vi "rsscope_core_global.vi"() -> ()   [LabVIEW 2018] (continued)
, "Data Type"=0, "Command"="BUS{SerialBus}:CXPI:IFS:MAX", "Access"=2, "Range Table"="RsScope_rngCXPIExpectedIFSMax", "Read Callback"="", "Write Callback"="", "Supported Models"="", "Instrument Options"="K76", "Flags"=0, "Help"="Sets the maximum for the inter-frame-space range.\n\nAvailable Repeated Capabilities:\nSerialBus: SB1, SB2, SB3, SB4\r\n\nRemote-control command(s):\nBUS<m>:CXPI:IFS:MAX"}, {"Level"=3, "Class Only"=TRUE, "Identifier"="", "Descriptive Name"="Decoding Results", "Data Type"=0, "Command"="", "Access"=0, "Range Table"="", "Read Callback"="", "Write Callback"="", "Supported Models"="", "Instrument Options"="", "Flags"=0, "Help"="Returns the CXPI decoding results."}, {"Level"=4, "Class Only"=FALSE, "Identifier"="RSSCOPE_ATTR_PROTOCOL_CXPI_FRAME_COUNT", "Descriptive Name"="Protocol CXPI Frame Count", "Data Type"=0, "Command"="BUS{SerialBus}:CXPI:RES:FCO?", "Access"=0, "Range Table"="", "Read Callback"="", "Write Callback"="", "Supported Models"="", "Instrument Options"="K76", "Flags"=0, "Help"="Returns the number of frames in the acquisition.\n\nAvailable Repeated Capabilities:\nSerialBus: SB1, SB2, SB3, SB4\r\n\nRemote-control command(s):\nBUS<m>:CXPI:RESult:FCOunt?"}, {"Level"=2, "Class Only"=TRUE, "Identifier"="", "Descriptive Name"="PCIe", "Data Type"=0, "Command"="", "Access"=0, "Range Table"="", "Read Callback"="", "Write Callback"="", "Supported Models"="", "Instrument Options"="", "Flags"=0, "Help"="R&S RTO-K72 is a firmware option that enables the R&S RTO to analyze Peripheral Component Interconnect Express (PCIe) signals encoded by the PCIe standard, generation 1 and 2."}, {"Level"=3, "Class Only"=FALSE, "Identifier"="RSSCOPE_ATTR_PROTOCOL_PCIE_GENERATION", "Descriptive Name"="Protocol PCIe Generation", "Data Type"=0, "Command"="BUS{SerialBus}:PCIE:GEN", "Access"=2, "Range Table"="RsScope_rngPCIeGeneration", "Read Callback"="", "Write Callback"="", "Supported Models"="", "Instrument Options"="", "Flags"=0, "Help"="Selects the generation of the PCIe technology.\n\nAvailable Repeated Capabilities:\nSerialBus: SB1, SB2, SB3, SB4\r\n\nRemote-control command(s):\nBUS<m>:PCIE:GEN"}, {"Level"=3, "Class Only"=FALSE, "Identifier"="RSSCOPE_ATTR_PROTOCOL_PCIE_LINK", "Descriptive Name"="Protocol PCIe Link", "Data Type"=0, "Command"="BUS{SerialBus}:PCIE:LNKW", "Access"=2, "Range Table"="RsScope_rngPCIeLink", "Read Callback"="", "Write Callback"="", "Supported Models"="", "Instrument Options"="K72", "Flags"=0, "Help"="Selects the link width, the number of lanes that are used for the transmission of the data.\n\nAvailable Repeated Capabilities:\nSerialBus: SB1, SB2, SB3, SB4\r\n\nRemote-control command(s):\nBUS<m>:PCIE:LNKW"}, {"Level"=3, "Class Only"=FALSE, "Identifier"="RSSCOPE_ATTR_PROTOCOL_PCIE_DESCRAMBLING", "Descriptive Name"="Protocol PCIe Descrambling", "Data Type"=3, "Command"="BUS{SerialBus}:PCIE:DSCR", "Access"=2, "Range Table"="", "Read Callback"="", "Write Callback"="", "Supported Models"="", "Instrument Options"="K72", "Flags"=0, "Help"="Enables descrambling of the data.\n\nAvailable Repeated Capabilities:\nSerialBus: SB1, SB2, SB3, SB4\r\n\nRemote-control command(s):\nBUS<m>:PCIE:DSCRambling"}, {"Level"=3, "Class Only"=FALSE, "Identifier"="RSSCOPE_ATTR_PROTOCOL_PCIE_FILTER_IDLE", "Descriptive Name"="Protocol PCIe Filter Idle", "Data Type"=3, "Command"="BUS{SerialBus}:PCIE:FIDL", "Access"=2, "Range Table"="", "Read Callback"="", "Write Callback"="", "Supported Models"="", "Instrument Options"="K72", "Flags"=0, "Help"="Enables the filtering of idle packets.\n\nAvailable Repeated Capabilities:\nSerialBus: SB1, SB2, SB3, SB4\r\n\nRemote-control command(s):\nBUS<m>:PCIE:FIDLe"}, {"Level"=3, "Class Only"=FALSE, "Identifier"="RSSCOPE_ATTR_PROTOCOL_PCIE_SHOW_MULTIPLE_LANES", "Descriptive Name"="Protocol PCIe Show Multiple Lanes", "Data Type"=3, "Command"="BUS{SerialBus}:PCIE:SML", "Access"=2, "Range Table"="", "Read Callback"="", "Write Callback"="", "Supported Models"="", "Instrument Options"="K72", "Flags"=0, "Help"="Enables the display of the result in multiple lanes.\n\nAvailable Repeated Capabilities:\nSerialBus: SB1, SB2, SB3, SB4\r\n\nRemote-control command(s):\nBUS<m>:PCIE:SMLanes"}, {"Level"=3, "Class Only"=TRUE, "Identifier"="", "Descriptive Name"="Lane", "Data Type"=0, "Command"="", "Access"=0, "Range Table"="", "Read Callback"="", "Write Callback"="", "Supported Models"="", "Instrument Options"="", "Flags"=0, "Help"="Class for Lane repcap."}, {"Level"=4, "Class Only"=FALSE, "Identifier"="RSSCOPE_ATTR_PROTOCOL_PCIE_SOURCE_LANE_ZERO", "Descriptive Name"="Protocol PCIe Source Lane Zero", "Data Type"=0, "Command"="BUS{SerialBus}:PCIE:LZER:SOUR", "Access"=2, "Range Table"="rsscope_rngProtocolWaveformSource", "Read Callback"="", "Write Callback"="", "Supported Models"="", "Instrument Options"="K72", "Flags"=0, "Help"="Sets the signal sources for Lane 0.\n\nAvailable Repeated Capabilities:\nSerialBus: SB1, SB2, SB3, SB4\r\n\nRemote-control command(s):\nBUS<m>:PCIE:LZER:SOURce"}, {"Level"=4, "Class Only"=FALSE, "Identifier"="RSSCOPE_ATTR_PROTOCOL_PCIE_SOURCE_LANE_ONE", "Descriptive Name"="Protocol PCIe Source Lane One", "Data Type"=0, "Command"="BUS{SerialBus}:PCIE:LONE:SOUR", "Access"=2, "Range Table"="rsscope_rngProtocolWaveformSource", "Read Callback"="", "Write Callback"="", "Supported Models"="", "Instrument Options"="K72", "Flags"=0, "Help"="Sets the signal sources for the corresponding logical lane.\n\nAvailable Repeated Capabilities:\nSerialBus: SB1, SB2, SB3, SB4\r\n\nRemote-control command(s):\nBUS<m>:PCIE:LONE:SOURce"}, {"Level"=4, "Class Only"=FALSE, "Identifier"="RSSCOPE_ATTR_PROTOCOL_PCIE_SOURCE_LANE_TWO", "Descriptive Name"="Protocol PCIe Source Lane Two", "Data Type"=0, "Command"="BUS{SerialBus}:PCIE:LTWO:SOUR", "Access"=2, "Range Table"="rsscope_rngProtocolWaveformSource", "Read Callback"="", "Write Callback"="", "Supported Models"="", "Instrument Options"="K72", "Flags"=0, "Help"="Sets the signal sources for the corresponding logical lane.\n\nAvailable Repeated Capabilities:\nSerialBus: SB1, SB2, SB3, SB4\r\n\nRemote-control command(s):\nBUS<m>:PCIE:LTWO:SOURce"}, {"Level"=4, "Class Only"=FALSE, "Identifier"="RSSCOPE_ATTR_PROTOCOL_PCIE_SOURCE_LANE_THREE", "Descriptive Name"="Protocol PCIe Source Lane Three", "Data Type"=0, "Command"="BUS{SerialBus}:PCIE:LTHR:SOUR", "Access"=2, "Range Table"="rsscope_rngProtocolWaveformSource", "Read Callback"="", "Write Callback"="", "Supported Models"="", "Instrument Options"="K72", "Flags"=0, "Help"="Sets the signal sources for the corresponding logical lane.\n\nAvailable Repeated Capabilities:\nSerialBus: SB1, SB2, SB3, SB4\r\n\nRemote-control command(s):\nBUS<m>:PCIE:LTHRee:SOURce"}, {"Level"=4, "Class Only"=FALSE, "Identifier"="RSSCOPE_ATTR_PROTOCOL_PCIE_THRESHOLD_LOW_LANE_ZERO", "Descriptive Name"="Protocol PCIe Threshold Low Lane Zero", "Data Type"=1, "Command"="BUS{SerialBus}:PCIE:LZER:THRL", "Access"=2, "Range Table"="RsScope_rngPCIeThreshold", "Read Callback"="", "Write Callback"="", "Supported Models"="", "Instrument Options"="K72", "Flags"=0, "Help"="Sets the lower threshold value for the respective lane.\n\nAvailable Repeated Capabilities:\nSerialBus: SB1, SB2, SB3, SB4\r\n\nRemote-control command(s):\nBUS<m>:PCIE:LZER:THRLow"}, {"Level"=4, "Class Only"=FALSE, "Identifier"="RSSCOPE_ATTR_PROTOCOL_PCIE_THRESHOLD_LOW_LANE_ONE", "Descriptive Name"="Protocol PCIe Threshold Low Lane One", "Data Type"=1, "Command"="BUS{SerialBus}:PCIE:LONE:THRL", "Access"=2, "Range Table"="RsScope_rngPCIeThreshold", "Read Callback"="", "Write Callback"="", "Supported Models"="", "Instrument Options"="K72", "Flags"=0, "Help"="Sets the lower threshold value for the respective lane.\n\nAvailable Repeated Capabilities:\nSerialBus: SB1, SB2, SB3, SB4\r\n\nRemote-control command(s):\nBUS<m>:PCIE:LONE:THRLow"}, {"Level"=4, "Class Only"=FALSE, "Identifier"="RSSCOPE_ATTR_PROTOCOL_PCIE_THRESHOLD_LOW_LANE_TWO", "Descriptive Name"="Protocol PCIe Threshold Low Lane Two", "Data Type"=1, "Command"="BUS{SerialBus}:PCIE:LTWO:THRL", "Access"=2, "Range Table"="RsScope_rngPCIeThreshold", "Read Callback"="", "Write Callback"="", "Supported Models"="", "Instrument Options"="K72", "Flags"=0, "Help"="Sets the lower threshold value for the respective lane.\n\nAvailable Repeated Capabilities:\nSerialBus: SB1, SB2, SB3, SB4\r\n\nRemote-control command(s):\nBUS<m>:PCIE:LTWO:THRLow"}, {"Level"=4, "Class Only"=FALSE, "Identifier"="RSSCOPE_ATTR_PROTOCOL_PCIE_THRESHOLD_LOW_LANE_THREE", "Descriptive Name"="Protocol PCIe Threshold Low Lane Three", "Data Type"=1, "Command"="BUS{SerialBus}:PCIE:LTHR:THRL", "Access"=2, "Range Table"="RsScope_rngPCIeThreshold", "Read Callback"="", "Write Callback"="", "Supported Models"="", "Instrument Options"="K72", "Flags"=0, "Help"="Sets the lower threshold value for the respective lane.\n\nAvailable Repeated Capabilities:\nSerialBus: SB1, SB2, SB3, SB4\r\n\nRemote-control command(s):\nBUS<m>:PCIE:LTHRee:THRLow"}, {"Level"=4, "Class Only"=FALSE, "Identifier"="RSSCOPE_ATTR_PROTOCOL_PCIE_THRESHOLD_HIGH_LANE_ZERO", "Descriptive Name"="Protocol PCIe Threshold High Lane Zero", "Data Type"=1, "Command"="BUS{SerialBus}:PCIE:LZER:THRH", "Access"=2, "Range Table"="RsScope_rngPCIeThreshold", "Read Callback"="", "Write Callback"="", "Supported Models"="", "Instrument Options"="K72", "Flags"=0, "Help"="Sets the high threshold value for the respective lane.\n\nAvailable Repeated Capabilities:\nSerialBus: SB1, SB2, SB3, SB4\r\n\nRemote-control command(s):\nBUS<m>:PCIE:LZER:THRHigh"}, {"Level"=4, "Class Only"=FALSE, "Identifier"="RSSCOPE_ATTR_PROTOCOL_PCIE_THRESHOLD_HIGH_LANE_ONE", "Descriptive Name"="Protocol PCIe Threshold High Lane One", "Data Type"=1, "Command"="BUS{SerialBus}:PCIE:LONE:THRH", "Access"=2, "Range Table"="RsScope_rngPCIeThreshold", "Read Callback"="", "Write Callback"="", "Supported Models"="", "Instrument Options"="K72", "Flags"=0, "Help"="Sets the high threshold value for the respective lane.\n\nAvailable Repeated Capabilities:\nSerialBus: SB1, SB2, SB3, SB4\r\n\nRemote-control command(s):\nBUS<m>:PCIE:LONE:THRHigh"}, {"Level"=4, "Class Only"=FALSE, "Identifier"="RSSCOPE_ATTR_PROTOCOL_PCIE_THRESHOLD_HIGH_LANE_TWO", "Descriptive Name"="Protocol PCIe Threshold High Lane Two", "Data Type"=1, "Command"="BUS{SerialBus}:PCIE:LTWO:THRH", "Access"=2, "Range Table"="RsScope_rngPCIeThreshold", "Read Callback"="", "Write Callback"="", "Supported Models"="", "Instrument Options"="K72", "Flags"=0, "Help"="Sets the high threshold value for the respective lane.\n\nAvailable Repeated Capabilities:\nSerialBus: SB1, SB2, SB3, SB4\r\n\nRemote-control command(s):\nBUS<m>:PCIE:LTWO:THRHigh"}, {"Level"=4, "Class Only"=FALSE, "Identifier"="RSSCOPE_ATTR_PROTOCOL_PCIE_THRESHOLD_HIGH_LANE_THREE", "Descriptive Name"="Protocol PCIe Threshold High Lane Three", "Data Type"=1, "Command"="BUS{SerialBus}:PCIE:LTHR:THRH", "Access"=2, "Range Table"="RsScope_rngPCIeThreshold", "Read Callback"="", "Write Callback"="", "Supported Models"="", "Instrument Options"="K72", "Flags"=0, "Help"="Sets the high threshold value for the respective lane.\n\nAvailable Repeated Capabilities:\nSerialBus: SB1, SB2, SB3, SB4\r\n\nRemote-control command(s):\nBUS<m>:PCIE:LTHRee:THRHigh"}, {"Level"=3, "Class Only"=TRUE, "Identifier"="", "Descriptive Name"="CDR", "Data Type"=0, "Command"="", "Access"=0, "Range Table"="", "Read Callback"="", "Write Callback"="", "Supported Models"="", "Instrument Options"="", "Flags"=0, "Help"="The process of clock data recovery (CDR) generates a reference clock from a highspeed serial data stream that is sent without a dedicated clock signal. The generated clock signal matches the frequency and is aligned to the phase of the data stream. The recovered clock can be used to sample the data stream and to obtain the sequence of transmitted bits."}, {"Level"=4, "Class Only"=FALSE, "Identifier"="RSSCOPE_ATTR_PROTOCOL_PCIE_CDR_NOMINAL_BITRATE", "Descriptive Name"="Protocol PCIe CDR Nominal Bitrate", "Data Type"=5, "Command"="BUS{SerialBus}:CDR:BITR", "Access"=2, "Range Table"="RsScope_rngPCIeCDRNominalBitrate", "Read Callback"="", "Write Callback"="", "Supported Models"="", "Instrument Options"="K72", "Flags"=0, "Help"="Sets the quiescent frequency of the PLL. It corresponds to the data rate of the data stream from which the clock is to be recovered.\n\nAvailable Repeated Capabilities:\nSerialBus: SB1, SB2, SB3, SB4\r\n\nRemote-control command(s):\nBUS<m>:CDR:BITRate"}, {"Level"=4, "Class Only"=FALSE, "Identifier"="RSSCOPE_ATTR_PROTOCOL_PCIE_CDR_PLL_ORDER", "Descriptive Name"="Protocol PCIe CDR PLL Order", "Data Type"=0, "Command"="BUS{SerialBus}:CDR:PLL:ORD", "Access"=2, "Range Table"="RsScope_rngPCIeCDRPLLOrder", "Read Callback"="", "Write Callback"="", "Supported Models"="", "Instrument Options"="K72", "Flags"=0, "Help"="Sets the order of the PLL: first or second order. PLL of higher order can compensate for more complex jitter behavior.\n\nAvailable Repeated Capabilities:\nSerialBus: SB1, SB2, SB3, SB4\r\n\nRemote-control command(s):\nBUS<m>:CDR:PLL:ORDer"}, {"Level"=4, "Class Only"=FALSE, "Identifier"="RSSCOPE_ATTR_PROTOCOL_PCIE_CDR_PLL_BANDWIDTH", "Descriptive Name"="Protocol PCIe CDR PLL Bandwidth", "Data Type"=1, "Command"="BUS{SerialBus}:CDR:PLL:BWID", "Access"=2, "Range Table"="", "Read Callback"="", "Write Callback"="", "Supported Models"="", "Instrument Options"="K72", "Flags"=0, "Help"="Sets the PLL bandwidth. It defines the part of the spectrum that the PLL can follow during synchronization. The PLL bandwidth is usually defined by the transmission standard.\n\nAvailable Repeated Capabilities:\nSerialBus: SB1, SB2, SB3, SB4\r\n\nRemote-control command(s):\nBUS<m>:CDR:PLL:BWIDth"}, {"Level"=4, "Class Only"=FALSE, "Identifier"="RSSCOPE_ATTR_PROTOCOL_PCIE_CDR_PLL_RELATIVE_BANDWIDTH", "Descriptive Name"="Protocol PCIe CDR PLL Relative Bandwidth", "Data Type"=1, "Command"="BUS{SerialBus}:CDR:PLL:RELB", "Access"=2, "Range Table"="RsScope_rngPCIeCDRPLLRelativeBandwidth", "Read Callback"="", "Write Callback"="", "Supported Models"="", "Instrument Options"="K72", "Flags"=0, "Help"="Sets the PLL bandwidth. It defines the part of the spectrum that the PLL can follow during synchronization. The PLL bandwidth is usually defined by the transmission standard.\n\nAvailable Repeated Capabilities:\nSerialBus: SB1, SB2, SB3, SB4\r\n\nRemote-control command(s):\nBUS<m>:CDR:PLL:RELBwidth"}, {"Level"=4, "Class Only"=FALSE, "Identifier"="RSSCOPE_ATTR_PROTOCOL_PCIE_CDR_PLL_DAMPING", "Descriptive Name"="Protocol PCIe CDR PLL Damping", "Data Type"=1, "Command"="BUS{SerialBus}:CDR:PLL:DAMP", "Access"=2, "Range Table"="RsScope_rngPCIeCDRPLLDamping", "Read Callback"="", "Write Callback"="", "Supported Models"="", "Instrument Options"="K72", "Flags"=0, "Help"="Sets the damping factor, which is only relevant for second order PLL.\n\nAvailable Repeated Capabilities:\nSerialBus: SB1, SB2, SB3, SB4\r\n\nRemote-control command(s):\nBUS<m>:CDR:PLL:DAMPing"}, {"Level"=4, "Class Only"=FALSE, "Identifier"="RSSCOPE_ATTR_PROTOCOL_PCIE_CDR_INITIAL_PHASE_SYNC", "Descriptive Name"="Protocol PCIe CDR Initial Phase Sync", "Data Type"=0, "Command"="BUS{SerialBus}:CDR:SYNC", "Access"=2, "Range Table"="RsScope_rngPCIeCDRInitialPhaseSync", "Read Callback"="", "Write Callback"="", "Supported Models"="", "Instrument Options"="K72", "Flags"=0, "Help"="Defines the phase reference for the first clock edge.\n\nAvailable Repeated Capabilities:\nSerialBus: SB1, SB2, SB3, SB4\r\n\nRemote-control command(s):\nBUS<m>:CDR:SYNC"}, {"Level"=4, "Class Only"=FALSE, "Identifier"="RSSCOPE_ATTR_PROTOCOL_PCIE_CDR_SELECTED_RESULTS", "Descriptive Name"="Protocol PCIe CDR Selected Results", "Data Type"=0, "Command"="BUS{SerialBus}:CDR:RES", "Access"=2, "Range Table"="RsScope_rngPCIeCDRSelectedResults", "Read Callback"="", "Write Callback"="", "Supported Models"="", "Instrument Options"="K72", "Flags"=0, "Help"="The PLL requires some time to synchronize to the phase of the data stream. You can select when the CDR algorithm returns clock edges.\n\nAvailable Repeated Capabilities:\nSerialBus: SB1, SB2, SB3, SB4\r\n\nRemote-control command(s):\nBUS<m>:CDR:RESults"}, {"Level"=3, "Class Only"=TRUE, "Identifier"="", "Descriptive Name"="DSP", "Data Type"=0, "Command"="", "Access"=0, "Range Table"="", "Read Callback"="", "Write Callback"="", "Supported Models"="", "Instrument Options"="", "Flags"=0, "Help"="You can enable and define the equalization techniques used for the equalization at the reciever side of the signal."}, {"Level"=4, "Class Only"=TRUE, "Identifier"="", "Descriptive Name"="DFE", "Data Type"=0, "Command"="", "Access"=0, "Range Table"="", "Read Callback"="", "Write Callback"="", "Supported Models"="", "Instrument Options"="", "Flags"=0, "Help"="Defines the settings of the decision feedback equalization (DFE). DFE correction is needed when the channel is distosrted."}, {"Level"=5, "Class Only"=FALSE, "Identifier"="RSSCOPE_ATTR_PROTOCOL_PCIE_DSP_DFE_ENABLED", "Descriptive Name"="Protocol PCIe DSP DFE Enabled", "Data Type"=3, "Command"="BUS{SerialBus}:PCIE:DFE:ENBL", "Access"=2, "Range Table"="", "Read Callback"="", "Write Callback"="", "Supported Models"="", "Instrument Options"="K72", "Flags"=0, "Help"="Enables the use of the decision feedback equalization for PCIe.\n\nAvailable Repeated Capabilities:\nSerialBus: SB1, SB2, SB3, SB4\r\n\nRemote-control command(s):\nBUS<m>:PCIE:DFE:ENBLe"}, {"Level"=5, "Class Only"=FALSE, "Identifier"="RSSCOPE_ATTR_PROTOCOL_PCIE_DSP_DFE_ESTIMATE_COEFFICIENTS_ENABLED", "Descriptive Name"="Protocol PCIe DSP DFE Estimate Coefficients Enabled", "Data Type"=3, "Command"="BUS{SerialBus}:PCIE:DFE:AUTO", "Access"=2, "Range Table"="", "Read Callback"="", "Write Callback"="", "Supported Models"="", "Instrument Options"="K72", "Flags"=0, "Help"="Enables the use of estimate coefficients\n\nAvailable Repeated Capabilities:\nSerialBus: SB1, SB2, SB3, SB4\r\n\nRemote-control command(s):\nBUS<m>:PCIE:DFE:AUTO"}, {"Level"=5, "Class Only"=FALSE, "Identifier"="RSSCOPE_ATTR_PROTOCOL_PCIE_DSP_DFE_COEFFICIENT", "Descriptive Name"="Protocol PCIe DSP DFE Coefficient", "Data Type"=1, "Command"="BUS{SerialBus}:PCIE:DFE:COEF", "Access"=2, "Range Table"="RsScope_rngDSPDFECoefficient", "Read Callback"="", "Write Callback"="", "Supported Models"="", "Instrument Options"="K72", "Flags"=0, "Help"="Sets the value of the coefficient for the DFE.\n\nAvailable Repeated Capabilities:\nSerialBus: SB1, SB2, SB3, SB4\r\n\nRemote-control command(s):\nBUS<m>:PCIE:DFE:COEFficient"}, {"Level"=5, "Class Only"=FALSE, "Identifier"="RSSCOPE_ATTR_PROTOCOL_PCIE_DSP_DFE_NUMBER_OF_TAPS", "Descriptive Name"="Protocol PCIe DSP DFE Number Of Taps", "Data Type"=0, "Command"="BUS{SerialBus}:PCIE:DFE:TCON", "Access"=2, "Range Table"="RsScope_rngDSPDFENumberOfTaps", "Read Callback"="", "Write Callback"="", "Supported Models"="", "Instrument Options"="K72", "Flags"=0, "Help"="Sets a number of taps for the decision feedback filter.\n\nAvailable Repeated Capabilities:\nSerialBus: SB1, SB2, SB3, SB4\r\n\nRemote-control command(s):\nBUS<m>:PCIE:DFE:TCONt"}, {"Level"=3, "Class Only"=TRUE, "Identifier"="", "Descriptive Name"="Decoding Results", "Data Type"=0, "Command"="", "Access"=0, "Range Table"="", "Read Callback"="", "Write Callback"="", "Supported Models"="", "Instrument Options"="", "Flags"=0, "Help"="Returns the PCIe decoding results."}, {"Level"=4, "Class Only"=FALSE, "Identifier"="RSSCOPE_ATTR_PROTOCOL_PCIE_PACKET_COUNT", "Descriptive Name"="Protocol PCIe Packet Count", "Data Type"=0, "Command"="BUS{SerialBus}:PCIE:RES:PCO?", "Access"=0, "Range Table"="", "Read Callback"="", "Write Callback"="", "Supported Models"="RTO|RTP", "Instrument Options"="K72", "Flags"=0, "Help"="Returns the packet count for the selected serial bus, i.e. the number of packets in the present acquisition.\n\nAvailable Repeated Capabilities:\nSerialBus: SB1, SB2, SB3, SB4\r\n\nRemote-control command(s):\nBUS<m>:PCIE:RESult:PCOunt?"}, {"Level"=4, "Class Only"=FALSE, "Identifier"="RSSCOPE_ATTR_PROTOCOL_PCIE_SELECTED_PACKET", "Descriptive Name"="Protocol PCIe Selected Packet", "Data Type"=0, "Command"="", "Access"=2, "Range Table"="", "Read Callback"="", "Write Callback"="", "Supported Models"="", "Instrument Options"="", "Flags"=0, "Help"="Sets the selector for the Packet repeated capability.\n\nAvailable Repeated Capabilities:\nNone\n\nRemote-control command(s):\n"}, {"Level"=4, "Class Only"=FALSE, "Identifier"="RSSCOPE_ATTR_PROTOCOL_PCIE_PACKET_BIT_RATE", "Descriptive Name"="Protocol PCIe Packet Bit Rate", "Data Type"=5, "Command"="BUS{SerialBus}:PCIE:RES:PACK<Packet>:BITR?", "Access"=0, "Range Table"="", "Read Callback"="rsscope_FormatPCIePacketRepCapInt64_ReadCallback.vi", "Write Callback"="rsscope_FormatPCIePacketRepCapInt64_WriteCallback.vi", "Supported Models"="", "Instrument Options"="", "Flags"=0, "Help"="Returns the bit rate of the selected packet.\n\nAvailable Repeated Capabilities:\nSerialBus: SB1, SB2, SB3, SB4\r\n\nRemote-control command(s):\nBUS<m>:PCIE:RESult:PACKet<n>:BITRate?"}, {"Level"=2, "Class Only"=TRUE, "Identifier"="", "Descriptive Name"="DDR", "Data Type"=0, "Command"="", "Access"=0, "Range Table"="", "Read Callback"="", "Write Callback"="", "Supported Models"="", "Instrument Options"="", "Flags"=0, "Help"="Double Data Rate memory (DDR) is a type of Synchronous Dynamic Random Access Memory (SDRAM). Option R&S RTO-K91"}, {"Level"=3, "Class Only"=FALSE, "Identifier"="RSSCOPE_ATTR_PROTOCOL_DDR_STANDARD", "Descriptive Name"="Protocol DDR Standard", "Data Type"=0, "Command"="BUS{SerialBus}:DDR:STAN", "Access"=2, "Range Table"="RsScope_rngDDRStandard", "Read Callback"="", "Write Callback"="", "Supported Models"="", "Instrument Options"="K91|K93", "Flags"=0, "Help"="Selects the DDR standard.\n\nAvailable Repeated Capabilities:\nSerialBus: SB1, SB2, SB3, SB4\r\n\nRemote-control command(s):\nBUS<m>:DDR:STANdard"}, {"Level"=3, "Class Only"=FALSE, "Identifier"="RSSCOPE_ATTR_PROTOCOL_DDR_DATA_SOURCE", "Descriptive Name"="Protocol DDR Data Source", "Data Type"=0, "Command"="BUS{SerialBus}:DDR:DATA:SOUR", "Access"=2, "Range Table"="rsscope_rngProtocolDDRSource", "Read Callback"="", "Write Callback"="", "Supported Models"="", "Instrument Options"="K91|K93", "Flags"=0, "Help"="Selects the source for the data output signal.\n\nAvailable Repeated Capabilities:\nSerialBus: SB1, SB2, SB3, SB4\r\n\nRemote-control command(s):\nBUS<m>:DDR:DATA:SOURce"}, {"Level"=3, "Class Only"=FALSE, "Identifier"="RSSCOPE_ATTR_PROTOCOL_DDR_DATA_THRESHOLD", "Descriptive Name"="Protocol DDR Data Threshold", "Data Type"=1, "Command"="BUS{SerialBus}:DDR:DATA:THR", "Access"=2, "Range Table"="RsScope_rngProtocolDDRThreshold", "Read Callback"="", "Write Callback"="", "Supported Models"="", "Instrument Options"="K91|K93", "Flags"=0, "Help"="Sets the threshold value for the digitization of the data line.\n\nAvailable Repeated Capabilities:\nSerialBus: SB1, SB2, SB3, SB4\r\n\nRemote-control command(s):\nBUS<m>:DDR:DATA:THReshold"}, {"Level"=3, "Class Only"=FALSE, "Identifier"="RSSCOPE_ATTR_PROTOCOL_DDR_DATA_HYSTERESIS", "Descriptive Name"="Protocol DDR Data Hysteresis", "Data Type"=1, "Command"="BUS{SerialBus}:DDR:DATA:HYST", "Access"=2, "Range Table"="RsScope_rngProtocolDDRHysteresis", "Read Callback"="", "Write Callback"="", "Supported Models"="", "Instrument Options"="K91|K93", "Flags"=0, "Help"="Sets a value for the hysteresis of the data.\n\nAvailable Repeated Capabilities:\nSerialBus: SB1, SB2, SB3, SB4\r\n\nRemote-control command(s):\nBUS<m>:DDR:DATA:HYSTeresis"}, {"Level"=3, "Class Only"=FALSE, "Identifier"="RSSCOPE_ATTR_PROTOCOL_DDR_STROBE_SOURCE", "Descriptive Name"="Protocol DDR Strobe Source", "Data Type"=0, "Command"="BUS{SerialBus}:DDR:STRB:SOUR", "Access"=2, "Range Table"="rsscope_rngProtocolDDRSource", "Read Callback"="", "Write Callback"="", "Supported Models"="", "Instrument Options"="K91|K93", "Flags"=0, "Help"="Selects the source for the strobe signal.\n\nAvailable Repeated Capabilities:\nSerialBus: SB1, SB2, SB3, SB4\r\n\nRemote-control command(s):\nBUS<m>:DDR:STRBe:SOURce"}, {"Level"=3, "Class Only"=FALSE, "Identifier"="RSSCOPE_ATTR_PROTOCOL_DDR_STROBE_THRESHOLD", "Descriptive Name"="Protocol DDR Strobe Threshold", "Data Type"=1, "Command"="BUS{SerialBus}:DDR:STRB:THR", "Access"=2, "Range Table"="RsScope_rngProtocolDDRThreshold", "Read Callback"="", "Write Callback"="", "Supported Models"="", "Instrument Options"="K91|K93", "Flags"=0, "Help"="Sets the threshold value for the digitization of the strobe line.\n\nAvailable Repeated Capabilities:\nSerialBus: SB1, SB2, SB3, SB4\r\n\nRemote-control command(s):\nBUS<m>:DDR:STRBe:THReshold"}, {"Level"=3, "Class Only"=FALSE, "Identifier"="RSSCOPE_ATTR_PROTOCOL_DDR_STROBE_HYSTERESIS", "Descriptive Name"="Protocol DDR Strobe Hysteresis", "Data Type"=1, "Command"="BUS{SerialBus}:DDR:STRB:HYST", "Access"=2, "Range Table"="RsScope_rngProtocolDDRHysteresis", "Read Callback"="", "Write Callback"="", "Supported Models"="", "Instrument Options"="K91|K93", "Flags"=0, "Help"="Sets a value for the hysteresis of the strobe.\n\nAvailable Repeated Capabilities:\nSerialBus: SB1, SB2, SB3, SB4\r\n\nRemote-control command(s):\nBUS<m>:DDR:STRBe:HYSTeresis"}, {"Level"=3, "Class Only"=TRUE, "Identifier"="", "Descriptive Name"="Decoding Results", "Data Type"=0, "Command"="", "Access"=0, "Range Table"="", "Read Callback"="", "Write Callback"="", "Supported Models"="", "Instrument Options"="", "Flags"=0, "Help"="Returns the DDR decoding results."}, {"Level"=4, "Class Only"=FALSE, "Identifier"="RSSCOPE_ATTR_PROTOCOL_DDR_FRAME_COUNT", "Descriptive Name"="Protocol DDR Frame Count", "Data Type"=0, "Command"="BUS{SerialBus}:DDR:RES:FCO?", "Access"=0, "Range Table"="", "Read Callback"="", "Write Callback"="", "Supported Models"="", "Instrument Options"="K91|K93", "Flags"=0, "Help"="Returns the number of decoded frames in the selected serial bus.\n\nAvailable Repeated Capabilities:\nSerialBus: SB1, SB2, SB3, SB4\r\n\nRemote-control command(s):\nBUS<m>:DDR:RESult:FCOunt?"}, {"Level"=4, "Class Only"=FALSE, "Identifier"="RSSCOPE_ATTR_PROTOCOL_DDR_SELECTED_FRAME", "Descriptive Name"="Protocol DDR Selected Frame", "Data Type"=0, "Command"="", "Access"=2, "Range Table"="", "Read Callback"="", "Write Callback"="", "Supported Models"="", "Instrument Options"="", "Flags"=0, "Help"="Sets selector repeated capability Frame.\n\nAvailable Repeated Capabilities:\nNone\n\nRemote-control command(s):\n"}, {"Level"=4, "Class Only"=FALSE, "Identifier"="RSSCOPE_ATTR_PROTOCOL_DDR_FRAME_STATUS", "Descriptive Name"="Protocol DDR Frame Status", "Data Type"=0, "Command"="BUS{SerialBus}:DDR:RES:FRAM<Frame>:STAT?", "Access"=0, "Range Table"="RsScope_rngDDRFrameStatus", "Read Callback"="rsscope_FormatDDRFrameRepCapInt32_ReadCallback.vi", "Write Callback"="", "Supported Models"="", "Instrument Options"="K91|K93", "Flags"=0, "Help"="Returns the status of the frame with the selected frame number (for the selected serial bus).\n\nAvailable Repeated Capabilities:\nSerialBus: SB1, SB2, SB3, SB4\r\n\nRemote-control command(s):\nBUS<m>:DDR:RESult:FRAMe<n>:STATe?"}, {"Level"=4, "Class Only"=FALSE, "Identifier"="RSSCOPE_ATTR_PROTOCOL_DDR_FRAME_START_TIME", "Descriptive Name"="Protocol DDR Frame Start Time", "Data Type"=1, "Command"="BUS{SerialBus}:DDR:RES:FRAM<Frame>:STAR?", "Access"=0, "Range Table"="", "Read Callback"="rsscope_FormatDDRFrameRepCapReal64_ReadCallback.vi", "Write Callback"="", "Supported Models"="", "Instrument Options"="K91|K93", "Flags"=0, "Help"="Returns the start time of the frame with the selected frame number (for the selected serial bus).\n\nAvailable Repeated Capabilities:\nSerialBus: SB1, SB2, SB3, SB4\r\n\nRemote-control command(s):\nBUS<m>:DDR:RESult:FRAMe<n>:STARt?"}, {"Level"=4, "Class Only"=FALSE, "Identifier"="RSSCOPE_ATTR_PROTOCOL_DDR_FRAME_STOP_TIME", "Descriptive Name"="Protocol DDR Frame Stop Time", "Data Type"=1, "Command"="BUS{SerialBus}:DDR:RES:FRAM<Frame>:STOP?", "Access"=0, "Range Table"="", "Read Callback"="rsscope_FormatDDRFrameRepCapReal64_ReadCallback.vi", "Write Callback"="", "Supported Models"="", "Instrument Options"="K91|K93", "Flags"=0, "Help"="Returns the stop time of the frame with the selected frame number (for the selected serial bus).\n\nAvailable Repeated Capabilities:\nSerialBus: SB1, SB2, SB3, SB4\r\n\nRemote-control command(s):\nBUS<m>:DDR:RESult:FRAMe<n>:STOP?"}, {"Level"=4, "Class Only"=FALSE, "Identifier"="RSSCOPE_ATTR_PROTOCOL_DDR_FRAME_TYPE", "Descriptive Name"="Protocol DDR Frame Type", "Data Type"=0, "Command"="BUS{SerialBus}:DDR:RES:FRAM<Frame>:TYPE?", "Access"=0, "Range Table"="RsScope_rngProtocolDDRFrameType", "Read Callback"="rsscope_FormatDDRFrameRepCapInt32_ReadCallback.vi", "Write Callback"="", "Supported Models"="", "Instrument Options"="K91|K93", "Flags"=0, "Help"="Returns the frame type for the selected serial bus and frame number.\n\nAvailable Repeated Capabilities:\nSerialBus: SB1, SB2, SB3, SB4\r\n\nRemote-control command(s):\nBUS<m>:DDR:RESult:FRAMe<n>:TYPE?"}, {"Level"=4, "Class Only"=FALSE, "Identifier"="RSSCOPE_ATTR_PROTOCOL_DDR_FRAME_NUMBER_OF_WORDS", "Descriptive Name"="Protocol DDR Frame Number Of Words", "Data Type"=0, "Command"="BUS{SerialBus}:DDR:RES:FRAM<Frame>:NWRD?", "Access"=0, "Range Table"="", "Read Callback"="rsscope_FormatDDRFrameRepCapInt32_ReadCallback.vi", "Write Callback"="", "Supported Models"="", "Instrument Options"="K91|K93", "Flags"=0, "Help"="Returns the number of words for the selected serial bus and frame number.\n\nAvailable Repeated Capabilities:\nSerialBus: SB1, SB2, SB3, SB4\r\n\nRemote-control command(s):\nBUS<m>:DDR:RESult:FRAMe<n>:NWRDs?"}, {"Level"=4, "Class Only"=FALSE, "Identifier"="RSSCOPE_ATTR_PROTOCOL_DDR_SELECTED_FIELD", "Descriptive Name"="Protocol DDR Selected Field", "Data Type"=0, "Command"="", "Access"=2, "Range Table"="", "Read Callback"="", "Write Callback"="", "Supported Models"="", "Instrument Options"="", "Flags"=0, "Help"="Sets selector repeated capability Field.\n\nAvailable Repeated Capabilities:\nNone\n\nRemote-control command(s):\n"}, {"Level"=4, "Class Only"=FALSE, "Identifier"="RSSCOPE_ATTR_PROTOCOL_DDR_FRAME_FIELD_STATUS", "Descriptive Name"="Protocol DDR Frame Field Status", "Data Type"=0, "Command"="BUS{SerialBus}:DDR:RES:FRAM<Frame>:FLD<Field>:STAT?", "Access"=0, "Range Table"="RsScope_rngDDRFrameStatus", "Read Callback"="rsscope_FormatDDRFieldRepCapInt32_ReadCallback.vi", "Write Callback"="", "Supported Models"="", "Instrument Options"="K91|K93", "Flags"=0, "Help"="Returns the status of the field with the selected field number within the frame with the selected frame number (for the selected serial bus).\n\nAvailable Repeated Capabilities:\nSerialBus: SB1, SB2, SB3, SB4\r\n\nRemote-control command(s):\nBUS<m>:DDR:RESult:FRAMe<n>:FLD<o>:STATus?"}, {"Level"=4, "Class Only"=FALSE, "Identifier"="RSSCOPE_ATTR_PROTOCOL_DDR_FRAME_FIELD_START_TIME", "Descriptive Name"="Protocol DDR Frame Field Start Time", "Data Type"=1, "Command"="BUS{SerialBus}:DDR:RES:FRAM<Frame>:FLD<Field>:STAR?", "Access"=0, "Range Table"="", "Read Callback"="rsscope_FormatDDRFieldRepCapReal64_ReadCallback.vi", "Write Callback"="", "Supported Models"="", "Instrument Options"="K91|K93", "Flags"=0, "Help"="Returns the start time of the field with the selected field number within the frame with the selected frame number (for the selected serial bus).\n\nAvailable Repeated Capabilities:\nSerialBus: SB1, SB2, SB3, SB4\r\n\nRemote-control command(s):\nBUS<m>:DDR:RESult:FRAMe<n>:FLD<o>:STARt?"}, {"Level"=4, "Class Only"=FALSE, "Identifier"="RSSCOPE_ATTR_PROTOCOL_DDR_FRAME_FIELD_STOP_TIME", "Descriptive Name"="Protocol DDR Frame Field Stop Time", "Data Type"=1, "Command"="BUS{SerialBus}:DDR:RES:FRAM<Frame>:FLD<Field>:STOP?", "Access"=0, "Range Table"="", "Read Callback"="rsscope_FormatDDRFieldRepCapReal64_ReadCallback.vi", "Write Callback"="", "Supported Models"="", "Instrument Options"="K91|K93", "Flags"=0, "Help"="Returns the stop time of the field with the selected field number within the frame with the selected frame number (for the selected serial bus).\n\nAvailable Repeated Capabilities:\nSerialBus: SB1, SB2, SB3, SB4\r\n\nRemote-control command(s):\nBUS<m>:DDR:RESult:FRAMe<n>:FLD<o>:STOP?"}, {"Level"=4, "Class Only"=FALSE, "Identifier"="RSSCOPE_ATTR_PROTOCOL_DDR_FRAME_FIELD_VALUE", "Descriptive Name"="Protocol DDR Frame Field Value", "Data Type"=0, "Command"="BUS{SerialBus}:DDR:RES:FRAM<Frame>:FLD<Field>:VAL?", "Access"=0, "Range Table"="", "Read Callback"="rsscope_FormatDDRFieldRepCapInt32_ReadCallback.vi", "Write Callback"="", "Supported Models"="", "Instrument Options"="K91|K93", "Flags"=0, "Help"="Returns the value of the field with the selected field number within the frame with the selected frame number (for the selected serial bus).\n\nAvailable Repeated Capabilities:\nSerialBus: SB1, SB2, SB3, SB4\r\n\nRemote-control command(s):\nBUS<m>:DDR:RESult:FRAMe<n>:FLD<o>:VAL?"}, {"Level"=4, "Class Only"=FALSE, "Identifier"="RSSCOPE_ATTR_PROTOCOL_DDR_FRAME_FIELD_FORMATTED_VALUE", "Descriptive Name"="Protocol DDR Frame Field Formatted Value", "Data Type"=2, "Command"="BUS{SerialBus}:DDR:RES:FRAM<Frame>:FLD<Field>:FVAL?", "Access"=0, "Range Table"="", "Read Callback"="rsscope_FormatDDRFieldRepCapString_ReadCallback.vi", "Write Callback"="", "Supported Models"="", "Instrument Options"="K91|K93", "Flags"=0, "Help"="Returns the formatted value of the field with the selected field number within the frame with the selected frame number (for the selected serial bus).\n\nAvailable Repeated Capabilities:\nSerialBus: SB1, SB2, SB3, SB4\r\n\nRemote-control command(s):\nBUS<m>:DDR:RESult:FRAMe<n>:FLD<o>:FVAL?"}, {"Level"=3, "Class Only"=TRUE, "Identifier"="", "Descriptive Name"="Eye Diagram", "Data Type"=0, "Command"="", "Access"=0, "Range Table"="", "Read Callback"="", "Write Callback"="", "Supported Models"="", "Instrument Options"="", "Flags"=0, "Help"="This class contains attributes and functions that provide eye diagram setup."}, {"Level"=4, "Class Only"=TRUE, "Identifier"="", "Descriptive Name"="Setup", "Data Type"=0, "Command"="", "Access"=0, "Range Table"="", "Read Callback"="", "Write Callback"="", "Supported Models"="", "Instrument Options"="", "Flags"=0, "Help"="Configure the source, the timing reference, and horizontal scale settings of the eye diagram. The vertical scale of the eye diagram is coupled to the vertical scale of the data source."}, {"Level"=5, "Class Only"=FALSE, "Identifier"="RSSCOPE_ATTR_EYE_DIAGRAM_STATE", "Descriptive Name"="Eye Diagram State", "Data Type"=3, "Command"="EYE{EyeDiagram}", "Access"=2, "Range Table"="", "Read Callback"="", "Write Callback"="", "Supported Models"="", "Instrument Options"="K91|K93", "Flags"=0, "Help"="Activates or deactivates the eye diagram.\n\nAvailable Repeated Capabilities:\nEyeDiagram: ED1, ED2, ED3, ED4\r\n\nRemote-control command(s):\nEYE<m>[:STATe]"}, {"Level"=5, "Class Only"=FALSE, "Identifier"="RSSCOPE_ATTR_EYE_DIAGRAM_SOURCE", "Descriptive Name"="Eye Diagram Source", "Data Type"=0, "Command"="EYE{EyeDiagram}:SOUR", "Access"=2, "Range Table"="rsscope_rngEyeDiagramSource", "Read Callback"="", "Write Callback"="", "Supported Models"="", "Instrument Options"="K91|K93", "Flags"=0, "Help"="Selects the waveform from which the eye diagram is generated (data source). For analog channels, peak detect, envelope, and average waveforms are not supported.\n\nAvailable Repeated Capabilities:\nEyeDiagram: ED1, ED2, ED3, ED4\r\n\nRemote-control command(s):\nEYE<m>:SOURce"}, {"Level"=5, "Class Only"=FALSE, "Identifier"="RSSCOPE_ATTR_EYE_DIAGRAM_BIT_RATE", "Descriptive Name"="Eye Diagram Bit Rate", "Data Type"=5, "Command"="BUS{EyeDiagram}:DDR:BITR", "Access"=2, "Range Table"="RsScope_rngEyeDiagramBitRate", "Read Callback"="", "Write Callback"="", "Supported Models"="", "Instrument Options"="K91|K93", "Flags"=0, "Help"="Declares the nominal bit rate of the data signal for the DDR eye diagram analysis.\n\nAvailable Repeated Capabilities:\nEyeDiagram: ED1, ED2, ED3, ED4\r\n\nRemote-control command(s):\nBUS<m>:DDR:BITRate"}, {"Level"=5, "Class Only"=FALSE, "Identifier"="RSSCOPE_ATTR_EYE_DIAGRAM_TIMING_REFERENCE_SOURCE", "Descriptive Name"="Eye Diagram Timing Reference Source", "Data Type"=0, "Command"="EYE{EyeDiagram}:TREF", "Access"=2, "Range Table"="rsscope_rngEyeDiagramSource", "Read Callback"="", "Write Callback"="", "Supported Models"="", "Instrument Options"="K91|K93", "Flags"=0, "Help"="Selects the waveform that is used to obtain the timing information required to slice the data source waveform.\n\nAvailable Repeated Capabilities:\nEyeDiagram: ED1, ED2, ED3, ED4\r\n\nRemote-control command(s):\nEYE<m>:TREFerence[:SOURce]"}, {"Level"=5, "Class Only"=FALSE, "Identifier"="RSSCOPE_ATTR_EYE_DIAGRAM_TIMING_REFERENCE_SLOPE", "Descriptive Name"="Eye Diagram Timing Reference Slope", "Data Type"=0, "Command"="EYE{EyeDiagram}:TREF:SLOP", "Access"=2, "Range Table"="RsScope_rngEyeDiagramTimingReferenceSlope", "Read Callback"="", "Write Callback"="", "Supported Models"="", "Instrument Options"="K91|K93", "Flags"=0, "Help"="Sets the edge on the timing reference waveform to define the timestamps for slicing the data waveform. A timestamp is set each time, when the selected slope of the timing waveform crosses the selected reference level.\n\nAvailable Repeated Capabilities:\nEyeDiagram: ED1, ED2, ED3, ED4\r\n\nRemote-control command(s):\nEYE<m>:TREFerence:SLOPe"}, {"Level"=5, "Class Only"=FALSE, "Identifier"="RSSCOPE_ATTR_EYE_DIAGRAM_TIME_REFERENCE_VERTICAL_REFERENCE_LEVEL", "Descriptive Name"="Eye Diagram Time Reference Vertical Reference Level", "Data Type"=0, "Command"="EYE{EyeDiagram}:TREF:LEV", "Access"=2, "Range Table"="RsScope_rngEyeDiagramVerticalReferenceLevel", "Read Callback"="", "Write Callback"="", "Supported Models"="", "Instrument Options"="K91|K93", "Flags"=0, "Help"="Sets the reference level on the timing reference waveform to define the timestamps for slicing the data waveform. A timestamp is set each time, when the selected slope of the timing waveform crosses the selected reference level.\n\nAvailable Repeated Capabilities:\nEyeDiagram: ED1, ED2, ED3, ED4\r\n\nRemote-control command(s):\nEYE<m>:TREFerence:LEVel"}, {"Level"=5, "Class Only"=FALSE, "Identifier"="RSSCOPE_ATTR_EYE_DIAGRAM_HORIZONTAL_SETTINGS_TIME_UNITS", "Descriptive Name"="Eye Diagram Horizontal Settings Time Units", "Data Type"=0, "Command"="EYE{EyeDiagram}:HOR", "Access"=2, "Range Table"="RsScope_rngEyeDiagramHorizontalSettingsTimeUnits", "Read Callback"="", "Write Callback"="", "Supported Models"="", "Instrument Options"="K91|K93", "Flags"=0, "Help"="Sets the method to define the horizontal scale of the eye diagram.\n\nAvailable Repeated Capabilities:\nEyeDiagram: ED1, ED2, ED3, ED4\r\n\nRemote-control command(s):\nEYE<m>:HORizontal[:UNIT]"}, {"Level"=5, "Class Only"=FALSE, "Identifier"="RSSCOPE_ATTR_EYE_DIAGRAM_HORIZONTAL_SETTINGS_TIME_RANGE", "Descriptive Name"="Eye Diagram Horizontal Settings Time Range", "Data Type"=1, "Command"="EYE{EyeDiagram}:HOR:ABS:RANG", "Access"=2, "Range Table"="RsScope_rngEyeDiagramHorizontalSettingsTimeRange", "Read Callback"="", "Write Callback"="", "Supported Models"="", "Instrument Options"="K91|K93", "Flags"=0, "Help"="Sets the time range that is covered by the eye diagram.\n\nAvailable Repeated Capabilities:\nEyeDiagram: ED1, ED2, ED3, ED4\r\n\nRemote-control command(s):\nEYE<m>:HORizontal:ABSolute:RANGe"}, {"Level"=5, "Class Only"=FALSE, "Identifier"="RSSCOPE_ATTR_EYE_DIAGRAM_HORIZONTAL_SETTINGS_TIME_POSITION", "Descriptive Name"="Eye Diagram Horizontal Settings Time Position", "Data Type"=1, "Command"="EYE{EyeDiagram}:HOR:ABS:POS", "Access"=2, "Range Table"="RsScope_rngEyeDiagramHorizontalSettingsTimePosition", "Read Callback"="", "Write Callback"="", "Supported Models"="", "Instrument Options"="K91|K93", "Flags"=0, "Help"="Sets the place of the zero point in the diagram, in seconds. The zero point is the alignment point on which the slice timestamps are superimposed.
